vi "Plot Update.vi"(6 "Control Ref Queue":T4, 8 "error in (no error)":errorcluster, 10 "Multiplot Representation In":T1, 11 "2D Plot.lvclass in":refnum<class "2D Plot.lvclass">) -> (0 "error out":errorcluster, 2 "Multiplot Representation Out":T1, 3 "2D Plot.lvclass out":refnum<class "2D Plot.lvclass">)   [LabVIEW 2020, in "2D Plot.lvclass"]
uses:
  <vilib>/Math Plots/2D Math Plots/2D Plot/2D Plot/2D Plot.lvclass
  <vilib>/Math Plots/2D Math Plots/2D Plot/2D Plot/Typedef/Multiplot Representation.ctl
  <vilib>/Math Plots/2D Math Plots/2D Plot/2D Plot/Typedef/Plot Representation.ctl
  <vilib>/Math Plots/2D Math Plots/2D Plot/2D Plot/Typedef/Range Cluster.ctl
  <vilib>/Math Plots/2D Math Plots/2D Plot/Action String/2DMathPlot Ctrl Act Queue.ctl
  <vilib>/Math Plots/2D Math Plots/2D Plot/Action String/2DMathPlot Ctrl Act Cluster.ctl
  <vilib>/Math Plots/2D Math Plots/2D Plot/Action String/2DMathPlot State Class.ctl
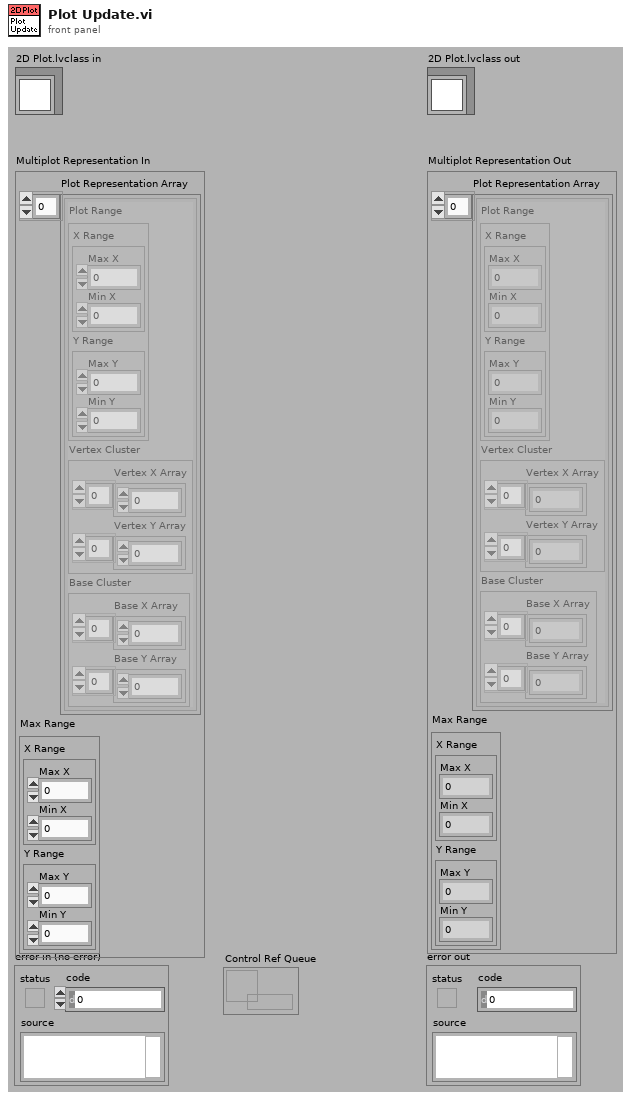
[diagram p1: front panel]
types:
  T1 = typedef "2D Plot.lvclass/Multiplot Representation.ctl" = cluster{"Plot Representation Array":T2[], "Max Range":T3}
  T2 = typedef "2D Plot.lvclass/Plot Representation.ctl" = cluster{"Plot Range":T3, "Vertex Cluster":cluster{"Vertex X Array":dbl[], "Vertex Y Array":dbl[]}, "Base Cluster":cluster{"Base X Array":dbl[], "Base Y Array":dbl[]}}
  T3 = typedef "2D Plot.lvclass/Range Cluster.ctl" = cluster{"X Range":cluster{"Max X":dbl, "Min X":dbl}, "Y Range":cluster{"Max Y":dbl, "Min Y":dbl}}
  T4 = typedef "2DMathPlot Ctrl Act Queue.ctl" = refnum<queue>
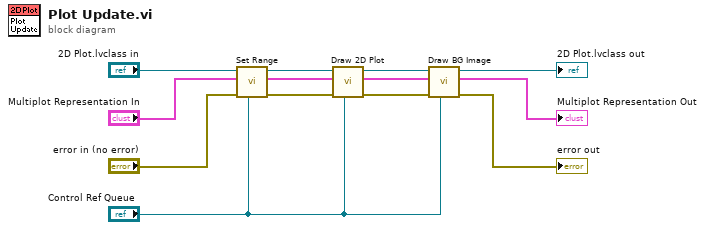
[diagram p0: block diagram]
diagram:
  n1 = call-dynamic "Set Range.vi"("Control Ref Queue"="Control Ref Queue", "error in (no error)"="error in (no error)", "Multiplot Representation In"="Multiplot Representation In", "2D Plot.lvclass in"="2D Plot.lvclass in") -> ("error out"=w12:errorcluster, "Multiplot Representation Out"=w11:T1, "2D Plot.lvclass out"=w8:refnum<class "2D Plot.lvclass">)  [unwired: 1 in, 4 out]
  n2 = call-dynamic "Draw 2D Plot.vi"("Control Ref Queue"="Control Ref Queue", "error in (no error)"=w12, "Multiplot Representation In"=w11, "2D Plot.lvclass in"=w8) -> ("error out"=w13:errorcluster, "Multiplot Representation Out"=w10:T1, "2D Plot.lvclass out"=w9:refnum<class "2D Plot.lvclass">)  [unwired: 1 in, 4 out]
  n3 = call-dynamic "Draw BG Image.vi"("Control Ref Queue"="Control Ref Queue", "error in (no error)"=w13, "Multiplot Representation In"=w10, "2D Plot.lvclass in"=w9) -> ("error out"=→"error out":errorcluster, "Multiplot Representation Out"=→"Multiplot Representation Out":T1, "2D Plot.lvclass out"=→"2D Plot.lvclass out":refnum<class "2D Plot.lvclass">)  [unwired: 5 out]
